vi "AlliGator Add New Gate to Dataset Images.vi"(7 "Buffer Image available?":bool, 8 "error in (no error)":errorcluster, 9 "Current Gate":i32, 10 "New Gate Image Refnum":T1, 11 "Dataset Images in":T2) -> (0 "error out":errorcluster, 1 "Current Gate (dup)":i32, 3 "Dataset Images out":T2)   [LabVIEW 2021, in "AlliGator Files.lvlib"]
doc: "Adds new gate image to dataset image structure."
uses:
  AlliGator Files.lvlib
  Internal Variables/AlliGator Gate Image Set.ctl
  <vilib>/vision/Image Controls.llb/IMAQ Image.ctl
  Internal Variables/AlliGator Internal Variables.lvlib
panel:
  # "see the AlliGator License on the block diagram (Ctrl+E or Window:Show Block Diagram)"
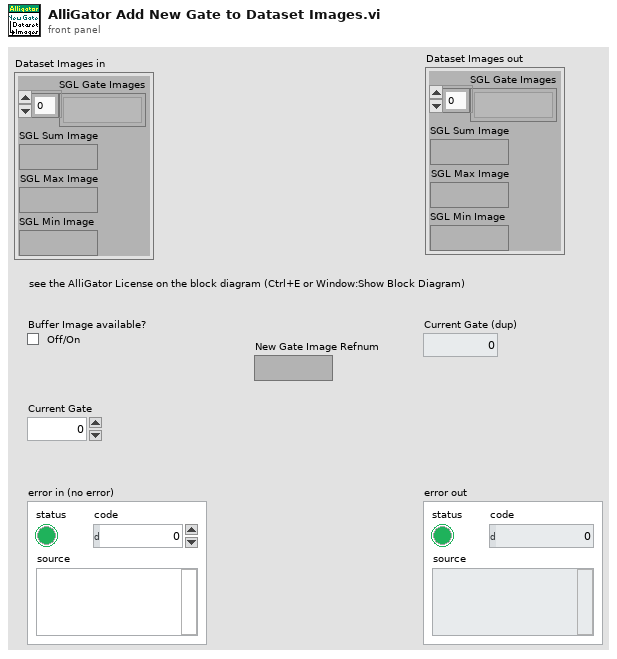
[diagram p1: front panel]
types:
  T1 = typedef "IMAQ Image.ctl" = refnum<image>
  T2 = typedef "AlliGator Internal Variables.lvlib/AlliGator Gate Image Set.ctl" = cluster{"SGL Gate Images":T1[], "SGL Sum Image":T1, "SGL Max Image":T1, "SGL Min Image":T1}
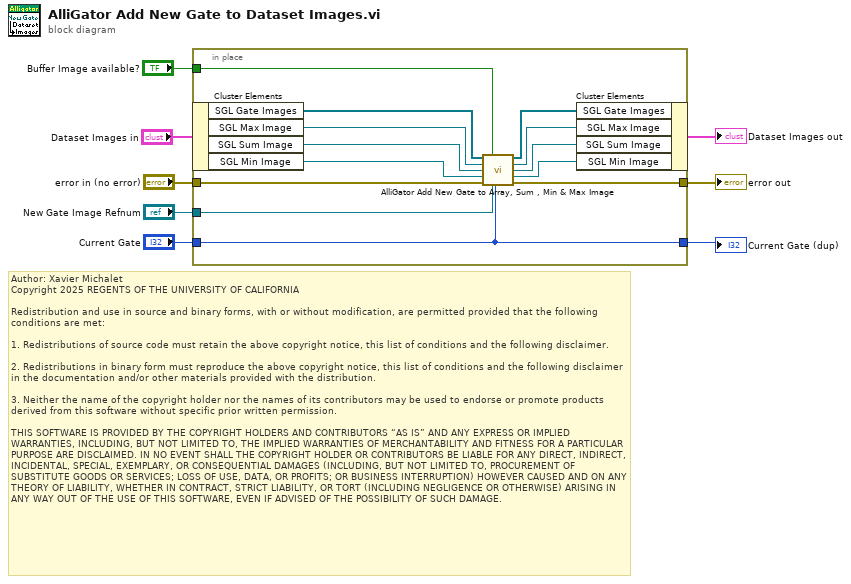
[diagram p0: block diagram]
diagram:
  # "Author: Xavier Michalet\nCopyright 2025 REGENTS OF THE UNIVERSITY OF CALIFORNIA\n\nRedistribution and use in source and binary forms, with or without modification, are permitted provided that the following conditions are met:\n\n1. Redistributions of source code must retain the above copyright notice, this list of conditions and the following disclaimer.\n\n2. Redistributions in binary form must reproduce the above copyright notice, this list of conditions and the following disclaimer in the documentation and/or other materials provided with the distribution.\n\n3. Neither the name of the copyright holder nor the names of its contributors may be used to endorse or promote products derived from this software without specific prior written permission.\n\nTHIS SOFTWARE IS PROVIDED BY THE COPYRIGHT HOLDERS AND CONTRIBUTORS “AS IS” AND ANY EXPRESS OR IMPLIED WARRANTIES, INCLUDING, BUT NOT LIMITED TO, THE IMPLIED WARRANTIES OF MERCHANTABILITY AND FITNESS FOR A PARTICULAR PURPOSE ARE DISCLAIMED. IN NO EVENT SHALL THE COPYRIGHT HOLDER OR CONTRIBUTORS BE LIABLE FOR ANY DIRECT, INDIRECT, INCIDENTAL, SPECIAL, EXEMPLARY, OR CONSEQUENTIAL DAMAGES (INCLUDING, BUT NOT LIMITED TO, PROCUREMENT OF SUBSTITUTE GOODS OR SERVICES; LOSS OF USE, DATA, OR PROFITS; OR BUSINESS INTERRUPTION) HOWEVER CAUSED AND ON ANY THEORY OF LIABILITY, WHETHER IN CONTRACT, STRICT LIABILITY, OR TORT (INCLUDING NEGLIGENCE OR OTHERWISE) ARISING IN ANY WAY OUT OF THE USE OF THIS SOFTWARE, EVEN IF ADVISED OF THE POSSIBILITY OF SUCH DAMAGE."
  n1 = in-place {
    in-place-border: "Buffer Image available?" -> [w21]
    in-place-border: "error in (no error)" -> [w20]
    in-place-border: "New Gate Image Refnum" -> [w19]
    in-place-border: [w18] -> w5
    in-place-border: "Current Gate" -> [w17]
    in-place-border: [w17] -> w3
    n2 = in-place-cluster #1("Dataset Images in") -> ("SGL Gate Images"=w16:T1[], "SGL Max Image"=w14:T1, "SGL Sum Image"=w12:T1, "SGL Min Image"=w10:T1)
    n3 = call "AlliGator Add New Gate to Array, Sum , Min & Max Image.vi"("SGL Gate Images in"=w16, "Buffer Image Available"=w21, "SGL Image Max in"=w14, "SGL Image Sum in"=w12, "SGL Image Min in"=w10, "error in (no error)"=w20, "Gate Image"=w19, "Current Gate"=w17) -> ("SGL Gate Images out"=w15:T1[], "SGL Image Max out"=w13:T1, "SGL Image Sum out"=w11:T1, "SGL Image Min out"=w9:T1, "error out"=w18:errorcluster)  [unwired: 3 in]
    n4 = in-place-cluster #1("SGL Gate Images"=w15, "SGL Max Image"=w13, "SGL Sum Image"=w11, "SGL Min Image"=w9) -> (→"Dataset Images out":T2)
  }
  "Current Gate (dup)" <- w3
  "error out" <- w5
